vi "Main.vi"() -> ()   [LabVIEW 2017, in "WebServiceImporter.lvlib" / "Main Panel.lvlib" / "Preview.lvlib"]
uses:
  <vilib>/Platform/WebService/Main Panel/Pages/Preview/Preview.lvlib
  <vilib>/Platform/WebService/Main Panel/Pages/Preview/Events/Events.lvlib
panel:
  in  "Panel":enum32{"Interface Frame", "Hidden Controls"}(tab)
  in  "Summary":string
  # "Summary"
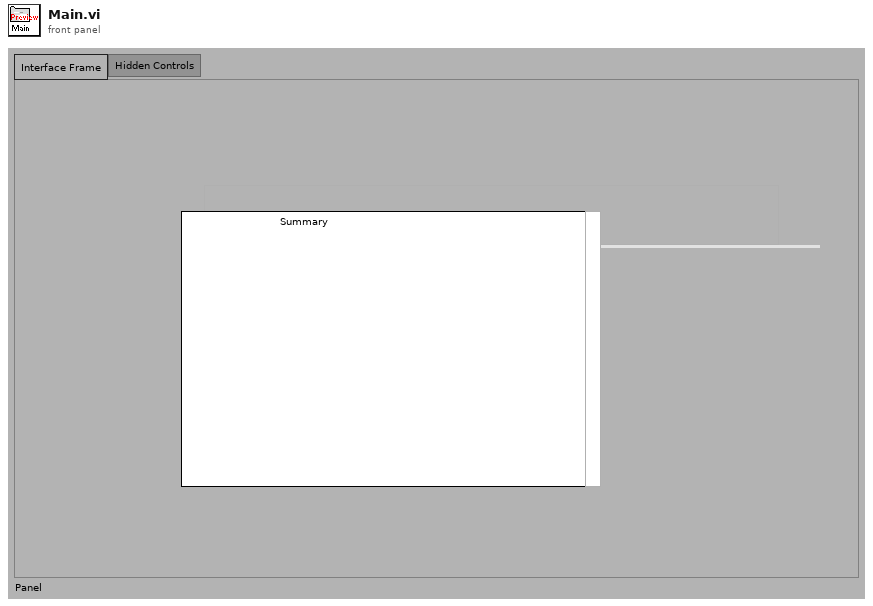
[diagram p1: front panel]
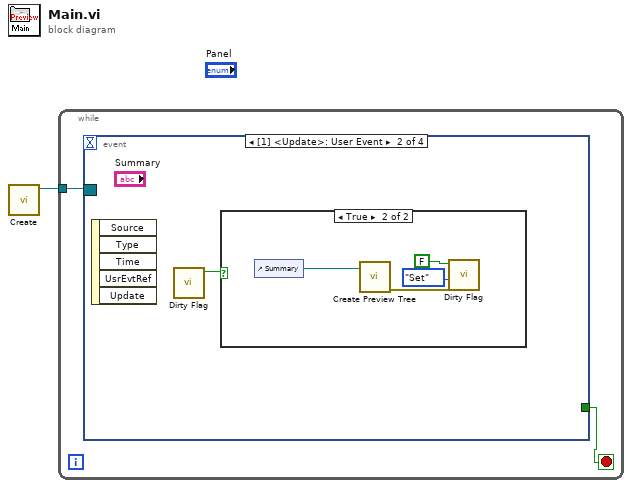
[diagram p0: block diagram]
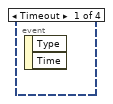
[diagram p2: hidden frame]
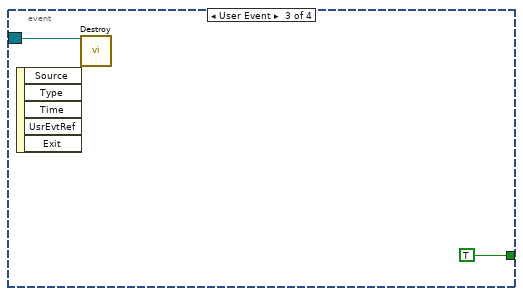
[diagram p4: hidden frame]
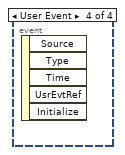
[diagram p5: hidden frame]
diagram:
  n1 = call <vilib>:"Create.vi"() -> ("Event Registration Refnum"=w1:refnum<event-registration>)  [unwired: 10 in, 1 out]
  n2 = while {
    tunnel: w1 -> [w3]
    stop <- w2 stop-if-true
    n3 = event shown="[1] <Update>: User Event" {
      selector: w3 -> [_ _ w9 _]
      dyn-events: _ -> [_ _ _ _]
      timeout: _ -> [_ _ _ _]
      tunnel: [_ _ TRUE _] -> w2
      event Timeout {
        n4 = event-data() -> ()  [unwired: 1 in, 2 out]
      }
      event User Event {
        n5 = event-data() -> ()  [unwired: 1 in, 5 out]
        n6 = call <vilib>:"Dirty Flag.vi"() -> ("Dirty (out)"=w4:bool)  [unwired: 10 in, 1 out]
        n7 = case shown="True" w4 {
          frame False {
          }
          frame True {
            n8 = control-ref of="Summary"() -> (w5:refnum<vi>)
            n9 = call <vilib>:"Create Preview Tree.vi"("Summary"=w5) -> ("error out"=w8:errorcluster)  [unwired: 10 in]
            n10 = call <vilib>:"Dirty Flag.vi"("error in (no error)"=w8, "Operation"=enum16{"Get", "Set"}."Set", "Dirty"=FALSE) -> ()  [unwired: 7 in, 2 out]
          }
        }
      }
      event User Event {
        n11 = event-data() -> ()  [unwired: 1 in, 5 out]
        n12 = call <vilib>:"Destroy.vi"("Event Registration Refnum"=w9) -> ()  [unwired: 10 in, 1 out]
      }
      event User Event {
        n13 = event-data() -> ()  [unwired: 1 in, 5 out]
      }
    }
  }
